vi "insert_element.vi"(10 "element":i32, 11 "array in":i32[](array[numeric])) -> (3 "array out":i32[](array[numeric]))   [LabVIEW 2015, in "PolyVIEW.lvclass"]
uses:
  PolyVIEW.lvclass
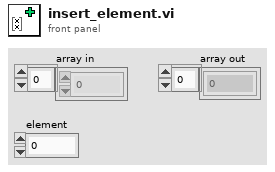
[diagram p1: front panel]
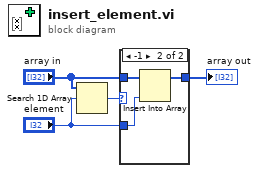
[diagram p0: block diagram]
diagram:
  n1 = Search 1D Array(1D array="array in", element="element") -> (index of element=w1:i32)  [unwired: 1 in]
  n2 = case shown="-1" w1 {
    tunnel: "array in" -> [w5 w8]
    tunnel: [w5 w7] -> w3
    tunnel: "element" -> [_ w6]
    frame Default {
    }
    frame -1 {
      n3 = Insert Into Array(array=w8, new element=w6) -> (w7:i32[])  [unwired: 1 in]
    }
  }
  "array out" <- w3
